vi "Get SMO PGSQL Log Paths.vi"(5 "getAll Cluster":variant, 7 "Paths":string, 8 "error in (no error)":errorcluster, 11 "Inst.FP in":refnum<class "Inst.FP.lvclass">) -> (0 "error out":errorcluster, 2 "Paths":string, 3 "Inst.FP out":refnum<class "Inst.FP.lvclass">)   [LabVIEW 2019, in "Inst.FP.lvclass"]
uses:
  Inst.FP.lvclass
  <userlib>/LevyLab/LV-Data/LV-Data.PG/LV-Data.PGSQL.lvclass
  <userlib>/LevyLab/Instrument Framework/SMOs/Configuration/Configuration.lvclass
  <userlib>/LevyLab/Instrument Framework/SMOs/Instrument/Instrument.lvclass
  Typedefs/Inst.FP.DefaultPGSQLPaths--Cluster.ctl
  Typedefs/Inst.FP.getAll--Cluster.ctl
  C:/Program Files (x86)/National Instruments/LabVIEW 2019/user.lib/LevyLab/Instrument Framework/Instrument Types/VSource/Instrument.VSource.lvclass
  C:/Program Files (x86)/National Instruments/LabVIEW 2019/user.lib/LevyLab/Instrument Framework/SMOs/Instrument/Instrument.lvclass
  C:/Program Files (x86)/National Instruments/LabVIEW 2019/vi.lib/JKI/JKI SMO/SMO/SMO.lvclass
  <userlib>/LevyLab/Instrument Framework/Instrument Types/VSource/Instrument.VSource.lvclass
  <userlib>/LevyLab/LV-Data/LV-Data.PG/API/Write Variable (one-row).vi
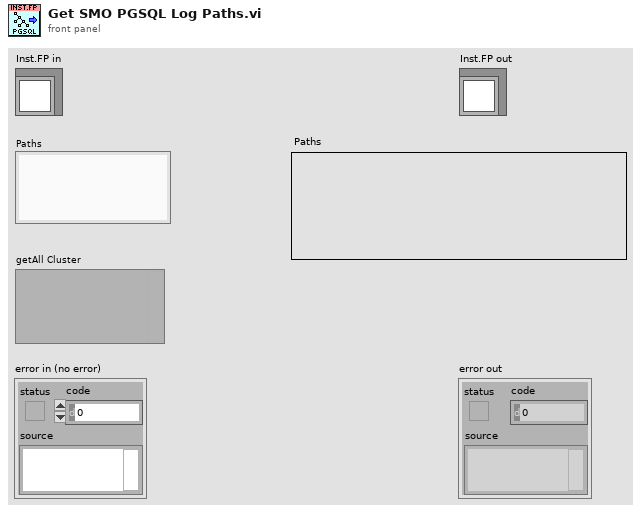
[diagram p1: front panel]
types:
  T1 = typedef "Inst.FP.lvclass/Inst.FP.DefaultPGSQLPaths--Cluster.ctl" = cluster{"CF":string, "MNK":string}
  T2 = typedef "Inst.FP.lvclass/Inst.FP.Type--Enum.ctl" = enum32{"Wet", "CF"}
  T3 = typedef "Inst.FP.lvclass/Inst.FP.getAll--Cluster.ctl" = cluster{"FP Data":dbl[], "MG Data":dbl[], "PT Data":dbl[], "Status Array":u32[], "Mode":string}
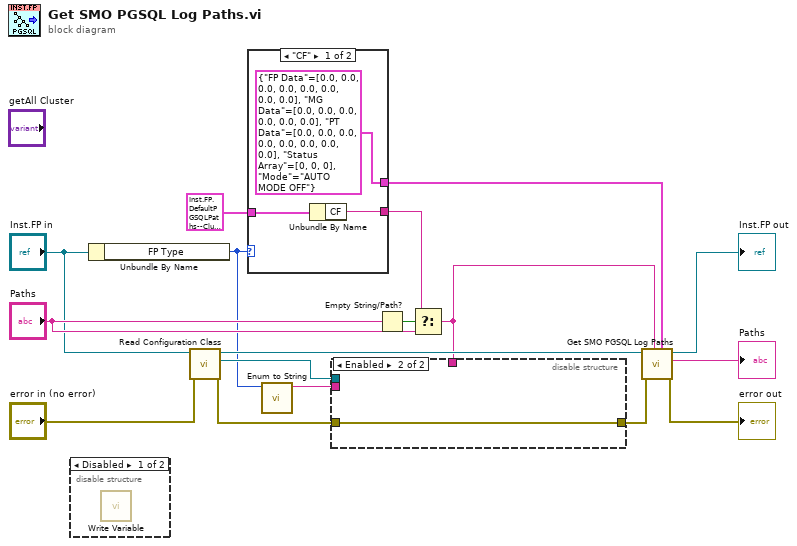
[diagram p0: block diagram]
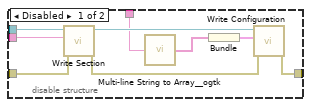
[diagram p2: hidden frame]
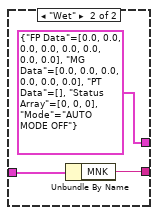
[diagram p3: hidden frame]
diagram:
  n1 = disable-structure shown="Disabled" {
    frame Disabled {
      n2 = call-poly <userlib>:"Write Variable.vi"() -> ()  [unwired: 8 in, 4 out]
    }
    frame Enabled {
    }
  }
  n3 = Unbundle By Name("Inst.FP in") -> ("FP Type"=w1:T2)
  n4 = call <userlib>:"Read Configuration Class.vi"("error in (no error)"="error in (no error)", "Instrument in"="Inst.FP in") -> ("error out"=w16:errorcluster, "Configuration"=w4:refnum<class "Configuration.lvclass">, "Instrument out"=w15:refnum<class "Inst.FP.lvclass">)  [unwired: 7 in]
  n5 = case shown="\"CF\"" w1 {
    tunnel: T1 {"CF"="llab_011:d000(Leiden CF FP--CF_FP_P1(mbar))\nllab_011:d001(Leiden CF FP--CF_FP_P2(mbar))\nllab_011:d002(Leiden CF FP--CF_FP_P3(mbar))\nllab_011:d003(Leiden CF FP--CF_FP_P4(mbar))\nllab_011:d004(Leiden CF FP--CF_FP_P5(mbar))\nllab_011:d005(Leiden CF FP--CF_FP_P6(mbar))\nllab_011:d006(Leiden CF FP--CF_FP_P7(mbar))\nllab_011:d007(Leiden CF FP--CF_FP_Flow())\nllab_011:d008(Leiden CF FP--CF_FP_MG0(mbar))\nllab_011:d009(Leiden CF FP--CF_FP_MG1(mbar))\nllab_011:d010(Leiden CF FP--CF_FP_MG2(mbar))\nllab_011:d011(Leiden CF FP--CF_FP_MG3(mbar))\nllab_011:d012(Leiden CF FP--CF_FP_MG4(mbar))\nllab_011:d013(Leiden CF FP--CF_FP_MG5(mbar))\nllab_011:d014(Leiden CF FP--CF_FP_PT_on())\nllab_011:d015(Leiden CF FP--CF_FP_PT_W_in_T(K))\nllab_011:d016(Leiden CF FP--CF_FP_PT_W_out_T(K))\nllab_011:d017(Leiden CF FP--CF_FP_PT_He_T(K))\nllab_011:d018(Leiden CF FP--CF_FP_PT_oil_T(K))\nllab_011:d019(Leiden CF FP--CF_FP_PT_P_Low(bar))\nllab_011:d020(Leiden CF FP--CF_FP_PT_P_High(bar))\nllab_011:d021(Leiden CF FP--CF_FP_PT_current(A))\nllab_011:d022(Leiden CF FP--CF_FP_state0())\nllab_011:d023(Leiden CF FP--CF_FP_state1())\nllab_011:d024(Leiden CF FP--CF_FP_state2())\nllab_011:v000(Leiden CF FP--CF_FP_STATE())", "MNK"="llab_016:d000(Leiden MNK Front Panel--MNK_FP_P1(mbar))\nllab_016:d001(Leiden MNK Front Panel--MNK_FP_P2(mbar))\nllab_016:d002(Leiden MNK Front Panel--MNK_FP_P3(mbar))\nllab_016:d003(Leiden MNK Front Panel--MNK_FP_P4(mbar))\nllab_016:d004(Leiden MNK Front Panel--MNK_FP_P5(mbar))\nllab_016:d005(Leiden MNK Front Panel--MNK_FP_P6(mbar))\nllab_016:d006(Leiden MNK Front Panel--MNK_FP_P7(mbar))\nllab_016:d013(Leiden MNK Front Panel--MNK_FP_Flow())\nllab_016:d007(Leiden MNK Front Panel--MNK_FP_MG0(mbar))\nllab_016:d008(Leiden MNK Front Panel--MNK_FP_MG1(mbar))\nllab_016:d009(Leiden MNK Front Panel--MNK_FP_MG2(mbar))\nllab_016:d010(Leiden MNK Front Panel--MNK_FP_MG3(mbar))\nllab_016:d011(Leiden MNK Front Panel--MNK_FP_MG4(mbar))\nllab_016:d012(Leiden MNK Front Panel--MNK_FP_MG5(mbar))\nllab_016:d014(Leiden MNK Front Panel--MNK_FP_state0())\nllab_016:d015(Leiden MNK Front Panel--MNK_FP_state1())\nllab_016:d016(Leiden MNK Front Panel--MNK_FP_state2())\nllab_016:v000(Leiden MNK Front Panel--MNK_FP_STATE())"} ("PGSQL Paths") -> [w20 w23]
    tunnel: [w19 w22] -> w12
    tunnel: [T3 {"FP Data"=[0.0, 0.0, 0.0, 0.0, 0.0, 0.0, 0.0, 0.0], "MG Data"=[0.0, 0.0, 0.0, 0.0, 0.0, 0.0], "PT Data"=[0.0, 0.0, 0.0, 0.0, 0.0, 0.0, 0.0, 0.0], "Status Array"=[0, 0, 0], "Mode"="AUTO MODE OFF"} ("GetAll") T3 {"FP Data"=[0.0, 0.0, 0.0, 0.0, 0.0, 0.0, 0.0, 0.0], "MG Data"=[0.0, 0.0, 0.0, 0.0, 0.0, 0.0], "PT Data"=[], "Status Array"=[0, 0, 0], "Mode"="AUTO MODE OFF"} ("GetAll")] -> w2
    frame "CF" {
      n6 = Unbundle By Name(w20) -> ("CF"=w19:string)
    }
    frame "Wet" {
      n7 = Unbundle By Name(w23) -> ("MNK"=w22:string)
    }
  }
  n8 = call <userlib>:"Enum to String.vi"("Command"=w1) -> ("Command"=w17:string)  [unwired: 9 in, 1 out]
  n9 = Empty String/Path?(string/path="Paths") -> (empty?=w13:bool)
  n10 = Select(t=w12, s=w13, f="Paths") -> (s? t:f=w11:string)
  n11 = disable-structure shown="Enabled" {
    disable-tunnel: w17 -> [w32 _]
    disable-tunnel: w16 -> [w28 w33]
    disable-tunnel: [w27 w33] -> w14
    disable-tunnel: w11 -> [w25 _]
    disable-tunnel: w4 -> [w24 _]
    frame Disabled {
      n12 = call <userlib>:"Write Section.vi"("error in (no error)"=w28, "Section"=w32, "Configuration in"=w24) -> ("error out"=w26:errorcluster, "Configuration out"=w31:refnum<class "Configuration.lvclass">)  [unwired: 7 in]
      n13 = call <userlib>:"Multi-line String to Array__ogtk.vi"("string"=w25) -> ("lines"=w29:string[])
      n14 = Bundle("lines"=w29) -> (w30:cluster{"lines":string[]})  [unwired: 1 in]
      n15 = call <userlib>:"Write Configuration.vi"("error in (no error)"=w26, "Variant"=w30, "Configuration in"=w31) -> ("error out"=w27:errorcluster)  [unwired: 7 in, 1 out]
    }
    frame Enabled {
    }
  }
  n16 = call-parent "Get SMO PGSQL Log Paths.vi"("getAll Cluster"=w2, "Default Paths"=w11, "error in (no error)"=w14, "Instrument in"=w15) -> ("error out"=→"error out":errorcluster, "Paths"=→"Paths":string, "Instrument out"=→"Inst.FP out":refnum<class "Inst.FP.lvclass">)  [unwired: 5 in]
